vi "Dashboard Main.vi"() -> ()   [LabVIEW 2015]
uses:
  <vilib>/Utility/miscctls.llb/LVRowAndColumnTypeDef.ctl
  <vilib>/event_ctls.llb/eventvkey.ctl
  <vilib>/Rock Robotics/WPI/Dashboard/WPI_DashboardLogging Global.vi
  <vilib>/Rock Robotics/Network Tables/NT Read Numeric Array.vi
  <vilib>/Rock Robotics/Network Tables/NT Read Boolean.vi
  <vilib>/Utility/config.llb/Write Key (String).vi
  <vilib>/Utility/config.llb/Write Key (I32).vi
  <vilib>/Utility/config.llb/NI_LVConfig.lvlib
panel:
  in  "TCP":refnum<k5>
  in  "Rec Mode":enum32{"Stop", "Record", "Playback"}(radio)
  in  "Vision":u16(ring) items=["Camera Off", "USB Camera SW", "USB Camera HW", "IP Camera"]
  out "Camera IP":string
  out "Image Message":string="Timeout in Camera Communications"
  in  "Dashboard Tab":T1(tab)
  out "Waveform Chart":dbl(graph)
  in  "Drive Mode":enum16{"Tank Drive", "Arcade Drive"}(ring)
  in  "Controller Mode":enum16{"X-Box Controller", "Joysticks"}(ring)
  in  "Select Auto":string(combo)
  out "NT Connection":bool
  in  "Camera Settings":T2={"Frame Rate"=30, "Compression"=30, "Size"=1} {"Frame Rate" scale=1.0..30.0; "Size" items=["640x480", "320x240", "160x120"]}
  out "MotorChart R":cluster{"Numeric":dbl, "Numeric":dbl}(graph)
  out "MotorChart L":T3(graph)
  out "MotorSliders R":cluster{"MotorSlide1":dbl, "MotorSlide2":dbl} {"MotorSlide2" scale=-1.0..1.0 scale format="%#_2e"; "MotorSlide1" scale=-1.0..1.0 scale format="%#_2e"}
  out "MotorSliders L":T4 {"MotorSlide4 2" scale=0.0..14.0 scale format="%#_2e"; "MotorSlide2" scale=-1.0..1.0 scale format="%#_2e"; "MotorSlide1" scale=-1.0..1.0 scale format="%#_2e"}
  out "Gyro":dbl(knob) scale=0.0..360.0
  out "JS1 Z":dbl(slide) scale=-1.0..1.0 scale format="%#_2e"
  out "JS1 Graph":cluster{"X":dbl, "Y":dbl}[](graph)
  out "JS1 Buttons":T5
  out "JS2 Z":dbl(slide) scale=-1.0..1.0 scale format="%#_2e"
  out "JS2 Graph":cluster{"X":dbl, "Y":dbl}[](graph)
  out "JS2 Buttons":T5
  out "Mode":T6(ring)=enum."Auto Disabled"
  in  "DB Camera Config":bool
  out "fps":dbl format="%#.1g"
  out "Mbps":dbl format="%#.1g"
  out "Mbps LED":bool
  out "Arm Angle":dbl(knob)
  out "Lower Switch":bool
  out "Upper Switch":bool
  out "Code Version":string
  out "Dashboard Version":string
  in  "DB/String 9":string
  in  "DB/String 8":string
  in  "DB/String 7":string
  in  "DB/String 6":string
  in  "DB/String 5":string
  in  "DB/String 4":string
  in  "DB/String 3":string
  in  "DB/String 2":string
  in  "DB/String 1":string
  in  "DB/String 0":string
  in  "DB/Slider 0":dbl(slide) scale=0.0..5.0
  in  "DB/Slider 1":dbl(slide) scale=0.0..5.0
  in  "DB/Slider 2":dbl(slide) scale=0.0..5.0
  in  "DB/Slider 3":dbl(slide) scale=0.0..5.0
  out "DB/LED 3":bool
  out "DB/LED 2":bool
  out "DB/LED 1":bool
  out "DB/LED 0":bool
  in  "DB/Button 3":bool
  in  "DB/Button 2":bool
  in  "DB/Button 1":bool
  in  "DB/Button 0":bool caption="New Name"
  in  "Test Slider":dbl(slide) scale=0.0..100.0 scale format="%#_3g"
  in  "On/Off":bool caption="Solenoid"
  in  "Test Name":u16(ring) items=["Select the test to run..."]
  in  "Test Tree":string(tree)
  in  "Motor":cluster{"Value":dbl, "Enable":bool} {"Value" scale=-1.0..1.0 scale format="%#_3g"}
  out "Progress":T7 {"Test Progress" scale=0.0..100.0}
  in  "Rev/Fwd":cluster{"Forward":bool, "Reverse":bool}
  in  "Test Ring":u16(ring) items=["Monochrome", "Color"]
  out "Cmd Status":string
  in  "Execute Command":bool
  in  "Command Params":string[][](table)
  in  "Command Selection":i32(listbox)
  in  "CheckList":i32(listbox)
  out "Tree":string(tree)
  out "Camera Image":T8(plugin-control)
  out "Background":bool
  # "Arm Angle"
  # "Left"
  # "Front"
  # "Right"
  # "Arm"
  # "Lower Switch"
  # "Upper Switch"
  # "Autonomous Mode"
  # "Controller Mode"
  # "Battery"
  # "Robot Code Version"
  # "Drive Mode"
  # "Dashboard Code Version"
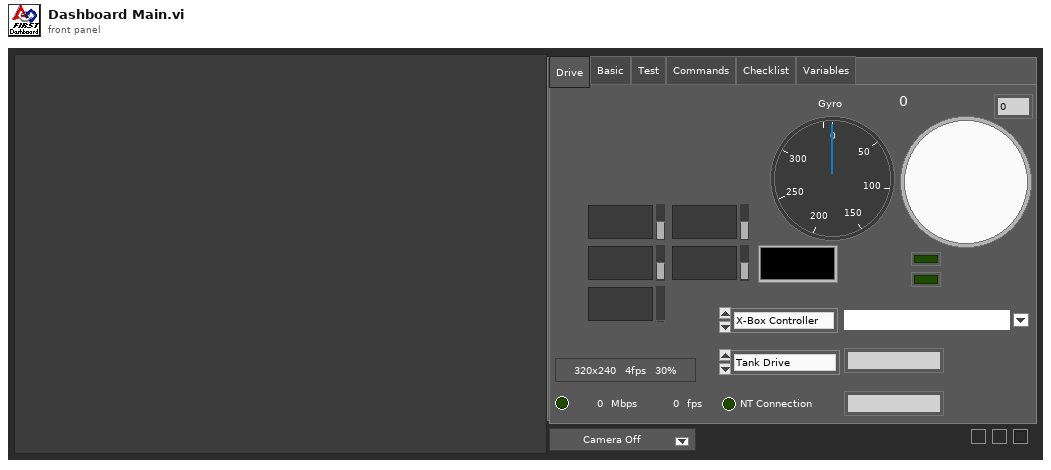
[diagram p1: front panel]
types:
  T1 = enum32{"Drive", "Basic", "Test", "Commands", "Checklist", "Variables"}
  T2 = cluster{"Frame Rate":i32, "Compression":i32, "Size":u16}
  T3 = cluster{"Numeric":dbl, "Numeric":dbl, "Battery V":dbl}
  T4 = cluster{"MotorSlide1":dbl, "MotorSlide2":dbl, "MotorSlide4 2":dbl}
  T5 = cluster{bool, bool, bool, bool, bool, bool, bool, bool, bool, bool, bool, bool}
  T6 = enum8{"Tele-Op Disabled", "Tele-Op Enabled", "Auto Disabled", "Auto Enabled", "Test Disabled", "Test Enabled", "Disconnected", "No Code", "E-Stop"}
  T7 = cluster{"Test Progress":u8, "Test Progress Text":string}
  T8 = typedef "IMAQ Image.ctl" = refnum<image>
  T9 = cluster{"IDs":cluster{"RPC field ID":u16, "Unique ID":u16}, "String":string}
  T10 = enum32{"Drive", "Basic", "Custom", "Test", "Checklist", "Variables"}
  T11 = typedef "Image Type" = u32
  T12 = cluster{"Camera Image":refnum<vi>, "Dashboard Tab":refnum<vi>, "Background":refnum<vi>, "Vision":refnum<vi>, "Rec Mode":refnum<vi>, "Test Slider":refnum<vi>, "On/Off ":refnum<vi>, "Test Ring":refnum<vi>, "Rev/Fwd":refnum<vi>, "Test Name":refnum<vi>, "Motor":refnum<vi>, "Progress":refnum<vi>, "CheckList":refnum<vi>, "Tree":refnum<vi>, "Test Tree":refnum<vi>, "Command Params":refnum<vi>, "Command Selection":refnum<vi>, "Execute Command":refnum<vi>, "Cmd Status":refnum<vi>}
  T13 = cluster{"Error Strings":string, "Disable Counts":cluster{u16, u16}, "Rail Faults":cluster{u16, u16, u16}, "Robot IP":string, "DB Mode":u8, "Event Info":cluster{"Name":string, "Type":u8, "Number":u16, "Replay":u8}, "Camera Addr":string}
  T14 = cluster{"Storage":cluster{"Disk Free":u64, "RAM Block":u32, "RAM free":u32}, "CPU Utilization":cluster{"CPU % ISR":sgl, "CPU % Time Crit":sgl, "CPU % Timed Str":sgl, "CPU % High":sgl, "CPU % Above":sgl, "CPU % Normal":sgl, "CPU % Low":sgl}, "CAN":cluster{"% Bus Utilization":sgl, "Bus Off Cnt":u32, "TX_FIFO Full Cnt":u32, "Receive Error Cnt":u8, "Transmit Error Cnt":u8}, "HID":cluster{"HID Outputs":u32, "Rumble Low":u16, "Rumble High":u16}[]}
  T15 = cluster{"Status bits":cluster{"Test Mode":bool, "Autonomous":bool, "Enabled":bool, "Code Start":bool, "Brownout":bool, "Reserved 2":bool, "Reserved 3":bool, "E-Stop":bool}, "Code Trace":cluster{"Disabled":bool, "TeleOp":bool, "Auto":bool, "Test":bool}, "Controller Type":enum16{"unknown", "cRIO", "roboRio"}, "Code?":enum16{"unknown", "noCode", "code"}, "Battery V":dbl}
  T16 = cluster{"Control Bits":cluster{"TestMode":bool, "Autonomous":bool, "Enabled":bool, "FMS Present":bool, bool, bool, bool, "E-Stop":bool}, "Team Station ":u8, "Countdown":sgl, "Joystick Values":cluster{"Axes":dbl[], "Buttons":bool[], "POVs":i16[]}[]}
  T17 = cluster{"Axes":dbl[], "Buttons":bool[], "POVs":i16[]}[]
  T18 = cluster{"Axes":dbl[], "Buttons":bool[], "POVs":i16[]}
  T19 = cluster{"Buttons[0]":bool, "Buttons[1]":bool, "Buttons[2]":bool, "Buttons[3]":bool, "Buttons[4]":bool, "Buttons[5]":bool, "Buttons[6]":bool, "Buttons[7]":bool, "Buttons[8]":bool, "Buttons[9]":bool, "Buttons[10]":bool, "Buttons[11]":bool}
  T20 = typedef "NI_LVConfig.lvlib/Config Data RefNum.ctl" = refnum<k1>
  T21 = cluster{"Operation":enum16{"Update", "Clear"}, "Color Box":u32}[]
  T22 = typedef "eventvkey.ctl" = enum16{"ASCII", "Enter", "Return", "Shift", "Ctrl", "Alt", "Cmd", "Opt", "Caps", "NumLock", "Clear", "Break", "Up", "Down", "Left", "Right", "Insert", "Delete", "Home", "End", "PageUp", "PageDown", "Escape", "Help", "Pause", "ScrollLock", "F1", "F2", "F3", "F4", "F5", "F6", "F7", "F8", "F9", "F10", "F11", "F12", "F13", "F14", "F15", "F16", "F17", "F18", "F19", "F20", "F21", "F22", "F23", "F24", "Play", "VolumeUp", "VolumeDown", "Mute", "Two Byte Char"}
  T23 = cluster{"Image Size":bool, "Image Type":bool, "Pixel Value":bool, "ROI Information":bool, "Zoom Factor":bool}
  T24 = enum8{"Enabled", "Disabled", "Disabled and Grayed Out"}
  T25 = cluster{"Operation":enum16{"Update", "Clear"}, "Color Box":u32}
  T26 = typedef "LVRowAndColumnTypeDef.ctl" = cluster{"Row":i32, "Column":i32}
  T27 = cluster{"Shift":bool, "Ctrl":bool, "Alt":bool, "Cmd":bool, "Opt":bool}
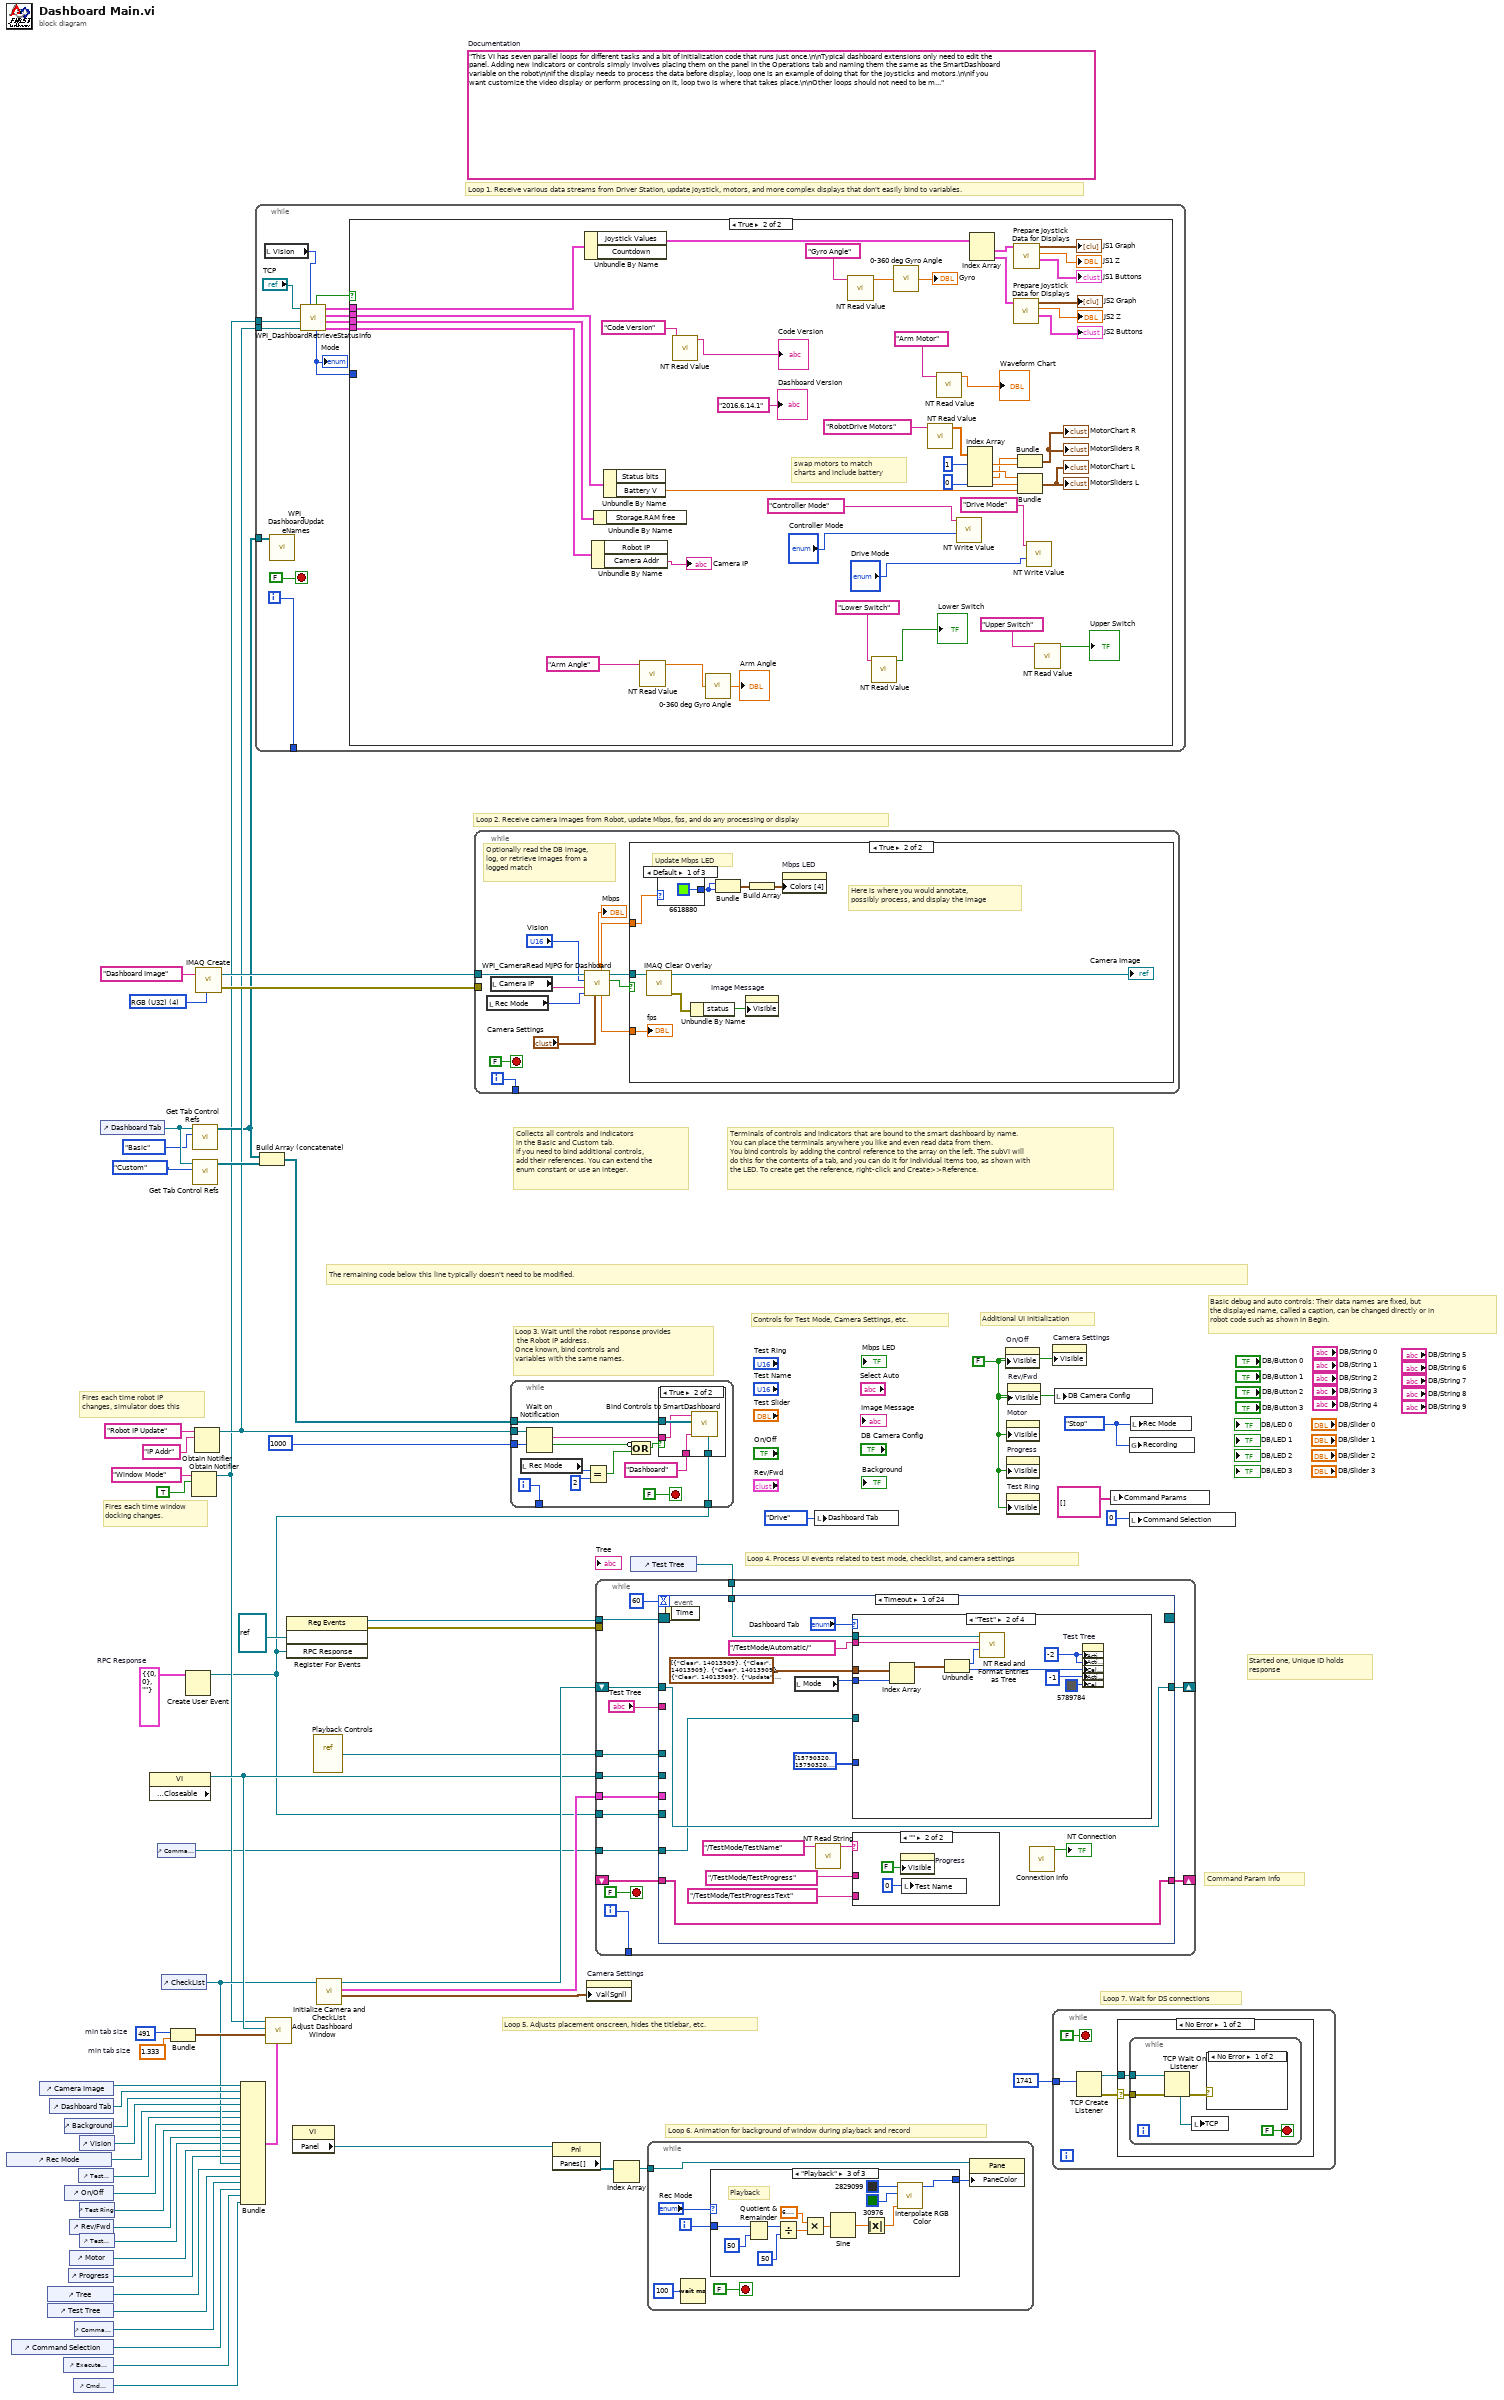
[diagram p0: block diagram]
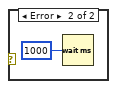
[diagram p2: hidden frame]
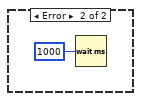
[diagram p3: hidden frame]
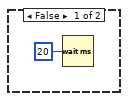
[diagram p4: hidden frame]
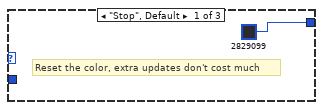
[diagram p5: hidden frame]
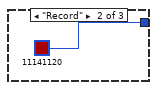
[diagram p6: hidden frame]
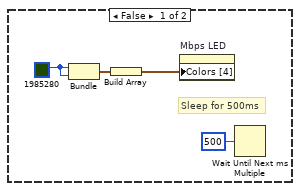
[diagram p8: hidden frame]
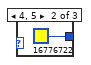
[diagram p9: hidden frame]
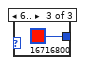
[diagram p10: hidden frame]
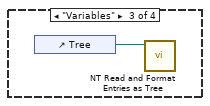
[diagram p12: hidden frame]
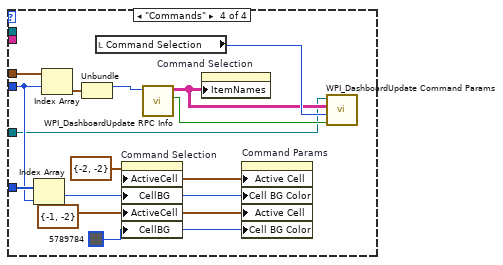
[diagram p13: hidden frame]
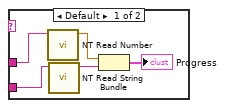
[diagram p14: hidden frame]
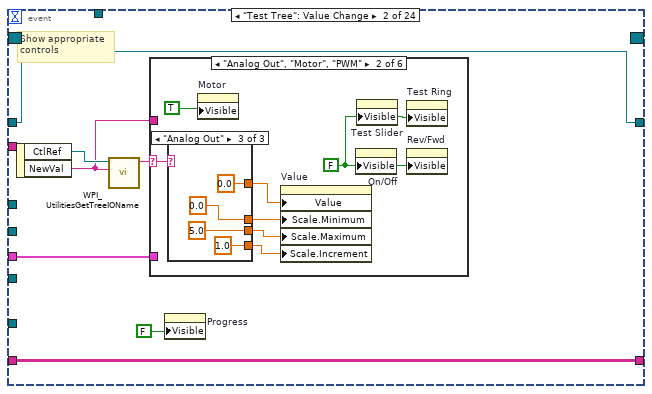
[diagram p15: hidden frame]
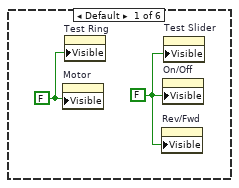
[diagram p16: hidden frame]
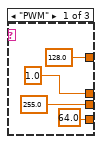
[diagram p17: hidden frame]
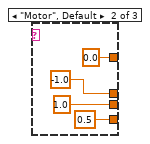
[diagram p18: hidden frame]
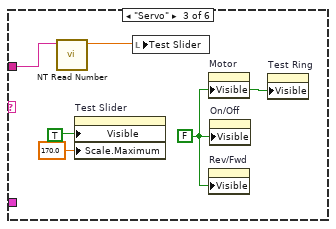
[diagram p19: hidden frame]
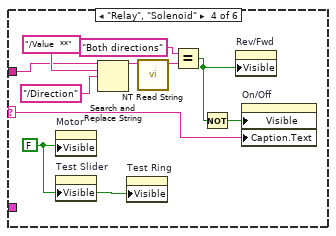
[diagram p20: hidden frame]
diagram:
  w8 = T9 {"IDs"={"RPC field ID"=0, "Unique ID"=0}, "String"=""}  # RPC Response
  w33 = 491  # min tab size
  w32 = 1.333  # min tab size
  w41 = enum32{"Stop", "Record", "Playback"}."Stop" ("Rec Mode")
  w15 = FALSE ("Visible")
  (unwired) "This VI has seven parallel loops for different tasks and a bit of initialization code that runs just once.\n\nTypical dashboard extensions only need to edit the panel. Adding new indicators or controls simply involves placing them on the panel in the Operations tab and naming them the same as the SmartDashboard variable on the robot\n\nIf the display needs to process the data before display, loop one is an example of doing that for the joysticks and motors.\n\nIf you want customize the video display or perform processing on it, loop two is where that takes place.\n\nOther loops should not need to be modified. They are pretty standard, and document the task they perform."  # Documentation
  w61 = T11 4 items=["Grayscale (U8)", "Grayscale (I16)", "Grayscale (SGL)", "Complex (CSG)", "RGB (U32)", "HSL (U32)", "RGB (U64)"] ("Image Type")
  # "Command Param Info"
  # "Started one, Unique ID holds\nresponse"
  # "Loop 7. Wait for DS connections"
  # "Basic debug and auto controls: Their data names are fixed, but\nthe displayed name, called a caption, can be changed directly or in\nrobot code such as shown in Begin."
  # "Controls for Test Mode, Camera Settings, etc."
  # "Additional UI Initialization"
  # "Loop 6. Animation for background of window during playback and record"
  # "Fires each time robot IP\nchanges, simulator does this"
  # "Fires each time window\ndocking changes."
  # "Collects all controls and indicators\nin the Basic and Custom tab.\nIf you need to bind additional controls,\nadd their references. You can extend the\nenum constant or use an integer."
  # "The remaining code below this line typically doesn't need to be modified."
  # "Loop 4. Process UI events related to test mode, checklist, and camera settings"
  # "Terminals of controls and indicators that are bound to the smart dashboard by name.\nYou can place the terminals anywhere you like and even read data from them.\nYou bind controls by adding the control reference to the array on the left. The subVI will\ndo this for the contents of a tab, and you can do it for individual items too, as shown with\nthe LED. To create get the reference, right-click and Create>>Reference."
  # "Loop 3. Wait until the robot response provides\n the Robot IP address.\nOnce known, bind controls and\nvariables with the same names."
  # "Loop 5. Adjusts placement onscreen, hides the titlebar, etc."
  # "Loop 1. Receive various data streams from Driver Station, update joystick, motors, and more complex displays that don't easily bind to variables."
  # "Loop 2. Receive camera images from Robot, update Mbps, fps, and do any processing or display"
  n1 = control-ref of="Rec Mode"() -> (w21:refnum<vi>)
  n2 = control-ref of="Command Selection"() -> (w7:refnum<vi>)
  n3 = control-ref of="Camera Image"() -> (w36:refnum<vi>)
  n4 = control-ref of="Tree"() -> (w25:refnum<vi>)
  n5 = control-ref of="Test Tree"() -> (w24:refnum<vi>)
  n6 = control-ref of="Dashboard Tab"() -> (w35:refnum<vi>)
  n7 = control-ref of="Execute Command"() -> (w9:refnum<vi>)
  n8 = control-ref of="Background"() -> (w30:refnum<vi>)
  n9 = control-ref of="On/Off"() -> (w19:refnum<vi>)
  n10 = control-ref of="Progress"() -> (w16:refnum<vi>)
  n11 = control-ref of="Rev/Fwd"() -> (w17:refnum<vi>)
  n12 = control-ref of="Motor"() -> (w22:refnum<vi>)
  n13 = control-ref of="Cmd Status"() -> (w3:refnum<vi>)
  n14 = control-ref of="Command Params"() -> (w10:refnum<vi>)
  n15 = control-ref of="Test Slider"() -> (w20:refnum<vi>)
  n16 = control-ref of="Vision"() -> (w34:refnum<vi>)
  n17 = control-ref of="Test Ring"() -> (w18:refnum<vi>)
  n18 = control-ref of="Test Name"() -> (w23:refnum<vi>)
  n19 = control-ref of="Dashboard Tab"() -> (w39:refnum<vi>)
  n20 = property class="VI" props=["Front Panel.Closeable"]() -> (reference out=w40:refnum<vi>)  [unwired: 2 in, 2 out]
  n21 = control-ref of="Command Params"() -> (w2:refnum<vi>)
  n22 = control-ref of="CheckList"() -> (w26:refnum<vi>)
  n23 = Bundle("min tab size"=w33, "min tab size"=w32) -> (w31:cluster{"min tab size":i32, "min tab size":dbl})  [unwired: 1 in]
  n24 = Create User Event(user event datatype=w8) -> (user event=w4:refnum<user-event>)  [unwired: 1 in, 1 out]
  n25 = Obtain Notifier(name (unnamed)="Window Mode", notification data type=TRUE) -> (notifier out=w12:refnum<notifier>)  [unwired: 2 in, 2 out]
  n26 = call <vilib>:"Get Tab Control Refs.vi"("Page Index"=T10."Basic" ("Dashboard Tab"), "TabControl in"=w39) -> ("ControlsOnPage"=w13:refnum<vi>[])  [unwired: 9 in]
  n27 = call <vilib>:"Get Tab Control Refs.vi"("Page Index"=T10."Custom" ("Dashboard Tab"), "TabControl in"=w39) -> ("ControlsOnPage"=w38:refnum<vi>[])  [unwired: 9 in]
  n28 = Obtain Notifier(name (unnamed)="Robot IP Update", notification data type="IP Addr" ("name (unnamed)")) -> (notifier out=w14:refnum<notifier>)  [unwired: 2 in, 2 out]
  n29 = call "IMAQ Create"("Image Name"="Dashboard Image", "Image Type"=w61) -> ("New Image"=w59:T8, "error out"=w58:errorcluster)  [unwired: 2 in, 1 out]
  n30 = Bundle("Camera Image"=w36, "Dashboard Tab"=w35, "Background"=w30, "Vision"=w34, "Rec Mode"=w21, "Test Slider"=w20, "On/Off"=w19, "Test Ring"=w18, "Rev/Fwd"=w17, "Test Name"=w23, "Motor"=w22, "Progress"=w16, "CheckList"=w26, "Tree"=w25, "Test Tree"=w24, "Command Params"=w10, "Command Selection"=w7, "Execute Command"=w9, "Cmd Status"=w3) -> (w27:T12)  [unwired: 1 in]
  n31 = while {
    tunnel: [w73] -> _
    tunnel: w14 -> [w67]
    tunnel: w13 -> [w66]
    tunnel: w12 -> [w62]
    i -> [w73]
    stop <- FALSE stop-if-true
    n32 = local read "Vision"() -> (w64:u16)
    n33 = call <vilib>:"WPI_DashboardUpdateNames.vi"("Controls on Tab"=w66) -> ()  [unwired: 11 in]
    n34 = call <vilib>:"WPI_DashboardRetrieveStatusInfo.vi"("Vision"=w64, "Binding Refnum"=w67, "Window Mode Notifier"=w62, "TCP Cnx"="TCP") -> ("Power and Errors"=w68:T13, "Robot Metrics"=w71:T14, "Status Info"=w72:T15, "Control Info"=w69:T16, "Robot Mode"=w65:T6, "Process?"=w70:bool)  [unwired: 2 in]
    "Mode" <- w65
    n35 = case shown="True" w70 {
      tunnel: w72 -> [_ w119]
      tunnel: w71 -> [_ w118]
      tunnel: w69 -> [_ w117]
      tunnel: w68 -> [_ w116]
      tunnel: w65 -> [_ _]
      frame False {
        n36 = Wait (ms)(milliseconds to wait=u32 20) -> ()  [unwired: 1 out]
      }
      frame True {
        # "swap motors to match\ncharts and include battery"
        n37 = Unbundle By Name(w117) -> ("Joystick Values"=w106:T17)  [unwired: 1 out]
        n38 = Unbundle By Name(w116) -> ("Camera Addr"=→"Camera IP":string)  [unwired: 1 out]
        n39 = Unbundle By Name(w118) -> ()  [unwired: 1 out]
        n40 = Unbundle By Name(w119) -> ("Battery V"=w107:dbl)  [unwired: 1 out]
        n41 = call-poly <vilib>:"NT Read Value.vi"("Name"="Arm Angle") -> ("Numeric"=w78:dbl)  [unwired: 9 in, 1 out]
        n42 = call-poly <vilib>:"NT Read Value.vi"("Name"="Code Version") -> ("String"=→"Code Version":string)  [unwired: 9 in, 1 out]
        n43 = call "0-360 deg Gyro Angle.vi"("Raw Angle"=w78) -> ("0-360 deg Angle"=→"Arm Angle":dbl)
        n44 = call-poly <vilib>:"NT Read Value.vi"("Name"="Gyro Angle") -> ("Numeric"=w76:dbl)  [unwired: 9 in, 1 out]
        n45 = call-poly <vilib>:"NT Read Value.vi"("Name"="Lower Switch") -> ("Boolean"=→"Lower Switch":bool)  [unwired: 9 in, 1 out]
        n46 = call "0-360 deg Gyro Angle.vi"("Raw Angle"=w76) -> ("0-360 deg Angle"=→"Gyro":dbl)
        n47 = call-poly <vilib>:"NT Read Value.vi"("Name"="RobotDrive Motors") -> ("Numeric Array"=w95:dbl[])  [unwired: 9 in, 1 out]
        n48 = call-poly <vilib>:"NT Read Value.vi"("Name"="Arm Motor") -> ("Numeric"=→"Waveform Chart":dbl)  [unwired: 9 in, 1 out]
        n49 = call-poly <vilib>:"NT Write Value.vi"("Numeric"="Controller Mode", "Name"="Controller Mode") -> ()  [unwired: 9 in, 1 out]
        n50 = Index Array(array=w95, index #1=1, index #4=0) -> (element #1=w111:dbl, element #2=w112:dbl, element #3=w110:dbl, element #4=w115:dbl)  [unwired: 2 in]
        n51 = Index Array(array=w106) -> (element #1=w105:T18, element #2=w100:T18)  [unwired: 2 in]
        n52 = call "Prepare Joystick Data for Displays.vi"("Joystick Values"=w100) -> ("Buttons"=→"JS2 Buttons":T19, "Z Axis"=→"JS2 Z":dbl, "Cartesian Data"=→"JS2 Graph":cluster{"X axis":dbl, "X axis":dbl}[])  [unwired: 8 in]
        n53 = call "Prepare Joystick Data for Displays.vi"("Joystick Values"=w105) -> ("Buttons"=→"JS1 Buttons":T19, "Z Axis"=→"JS1 Z":dbl, "Cartesian Data"=→"JS1 Graph":cluster{"X axis":dbl, "X axis":dbl}[])  [unwired: 8 in]
        n54 = Bundle("Numeric"=w110, "Numeric"=w111) -> (→"MotorChart R" →"MotorSliders R":cluster{"Numeric":dbl, "Numeric":dbl})  [unwired: 1 in]
        n55 = Bundle("Numeric"=w112, "Numeric"=w115, "Battery V"=w107) -> (→"MotorChart L" →"MotorSliders L":T3)  [unwired: 1 in]
        n56 = call-poly <vilib>:"NT Write Value.vi"("Numeric"="Drive Mode", "Name"="Drive Mode") -> ()  [unwired: 9 in, 1 out]
        n57 = call-poly <vilib>:"NT Read Value.vi"("Name"="Upper Switch") -> ("Boolean"=→"Upper Switch":bool)  [unwired: 9 in, 1 out]
        "Dashboard Version" <- "2016.6.14.1" ("Dashboard Version")
      }
    }
  }
  n58 = Build Array (concatenate)(w13, w38) -> (w37:refnum<vi>[])
  n59 = call "Adjust Dashboard Window.vi"("Sizing Refnums"=w27, "Size Constraints"=w31, "VI"=w40, "WIn Mode"=w12) -> ()  [unwired: 8 in]
  n60 = register-events(refnum<vi> refnum, w4) -> (reference out=w45:refnum<event-registration>, error out=w44:errorcluster)  [unwired: 2 in]
  n61 = property class="VI"() -> ("Panel"=w48:refnum<vi>)  [unwired: 2 in, 2 out]
  n62 = vi-ref "Playback Controls.vi"() -> (w46:refnum<vi>)
  n63 = call "Initialize Camera and CheckList.vi"("ListBox in"=w26) -> ("Cluster"=w52:cluster{"value":i32, "value":i32, "index":i32}, "Array"=w53:cluster{string[]}[], "File Refnum"=w51:T20)  [unwired: 8 in]
  n64 = while {
    tunnel: w59 -> [w128]
    tunnel: w58 -> [_]
    tunnel: [w129] -> _
    i -> [w129]
    stop <- FALSE stop-if-true
    # "Optionally read the DB image,\nlog, or retrieve images from a\nlogged match"
    n65 = local read "Rec Mode"() -> (w123:enum32{"Stop", "Record", "Playback"})
    n66 = local read "Camera IP"() -> (w121:string)
    n67 = call <vilib>:"WPI_CameraRead MJPG for Dashboard.vi"("Camera Settings"="Camera Settings", "Rec Mode"=w123, "Camera IP"=w121, "Camera Mode"="Vision", "Refnum in"=w128) -> ("Active"=w126:bool, "Refnum out"=w127:T8, "FPS"=w125:dbl, "Bandwidth (Mbps)"=w120:dbl)  [unwired: 3 in]
    "Mbps" <- w120
    n68 = case shown="True" w126 {
      tunnel: w127 -> [_ w138]
      tunnel: w120 -> [_ w137]
      tunnel: w125 -> [_ w135]
      frame False {
        w131 = u32 1985280 ("Color Box")
        # "Sleep for 500ms"
        n69 = Bundle("Color Box"=w131, "Color Box"=w131) -> (w133:cluster{"Color Box":u32, "Color Box":u32})  [unwired: 1 out]
        n70 = Build Array(w133) -> (w132:cluster{"Color Box":u32, "Color Box":u32}[])
        n71 = property on="Mbps LED" class="Bool (strict)"("Colors [4]"=w132) -> ()  [unwired: 2 in, 2 out]
        n72 = Wait Until Next ms Multiple(millisecond multiple=u32 500) -> ()  [unwired: 1 out]
      }
      frame True {
        # "Here is where you would annotate,\npossibly process, and display the image"
        # "Update Mbps LED"
        n73 = call "IMAQ Clear Overlay"("Image"=w138) -> ("error out"=w142:errorcluster, "Image Out"=→"Camera Image":T8)  [unwired: 2 in, 7 out]
        n74 = case shown="Default" w137 {
          tunnel: [u32 6618880 ("Color Box") u32 16776722 ("Color Box") u32 16716800 ("Color Box")] -> w139
          frame Default {
          }
          frame 4, 5 {
          }
          frame 6.. {
          }
        }
        n75 = Unbundle By Name(w142) -> ("status"=w143:bool)
        n76 = Bundle("Color Box"=w139, "Color Box"=w139) -> (w141:cluster{"Color Box":u32, "Color Box":u32})  [unwired: 1 out]
        n77 = property on="Image Message" class="Str"("Visible"=w143) -> ()  [unwired: 2 in, 2 out]
        n78 = Build Array(w141) -> (w140:cluster{"Color Box":u32, "Color Box":u32}[])
        n79 = property on="Mbps LED" class="Bool (strict)"("Colors [4]"=w140) -> ()  [unwired: 2 in, 2 out]
        "fps" <- w135
      }
    }
  }
  n80 = while {
    tunnel: w37 -> [w159]
    tunnel: w14 -> [w157]
    tunnel: [w155] -> _
    tunnel: u32 1000 ("milliseconds to wait") -> [w154]
    tunnel: w4 -> [w147]
    i -> [w155]
    stop <- FALSE stop-if-true
    n81 = local read "Rec Mode"() -> (w150:enum32{"Stop", "Record", "Playback"})
    n82 = Wait on Notification(notifier=w157, timeout in ms (-1)=w154) -> (notification=w156:string, timed out?=w152:bool)  [unwired: 2 in, 2 out]
    n83 = Equal?(x=w150, y=u16 2 ("Rec Mode")) -> (x = y?=w151:bool)
    n84 = Compound Arithmetic op=OR(invert w152, w151) -> (w153:bool)
    n85 = case shown="True" w153 {
      tunnel: w159 -> [_ w163]
      tunnel: w156 -> [_ w162]
      tunnel: "Dashboard" -> [_ w161]
      tunnel: w147 -> [_ w160]
      frame False {
      }
      frame True {
        n86 = call <vilib>:"Bind Controls to SmartDashboard.vi"("RPC ref"=w160, "Client Name"=w161, "Bound Control Refs"=w163, "Server IP Address"=w162) -> ()  [unwired: 8 in]
      }
    }
  }
  n87 = property class="Pnl"(reference=w48) -> ("Panes[]"=w49:refnum<vi>[])  [unwired: 1 in, 2 out]
  n88 = property on="Camera Settings" class="Clust (strict)"("Val(Sgnl)"=w52) -> ()  [unwired: 2 in, 2 out]
  n89 = Index Array(array=w49) -> (element=w47:refnum<vi>)  [unwired: 1 in]
  n90 = control-ref of="Test Tree"() -> (w50:refnum<vi>)
  n91 = while {
    tunnel: w53 -> [w175]
    shift-right: [w174] -> _
    shift-left: w51 -> [w173]
    tunnel: [w172] -> _
    tunnel: w50 -> [w171]
    tunnel: w46 -> [w170]
    tunnel: w45 -> [w169]
    tunnel: w44 -> [_]
    tunnel: w40 -> [w168]
    tunnel: w4 -> [w167]
    tunnel: w2 -> [w166]
    shift-right: [w165] -> _
    shift-left: _ -> [w164]
    i -> [w172]
    stop <- FALSE stop-if-true
    n92 = event shown="[0] Timeout" {
      selector: w169 -> [_ _ _ _ _ _ _ _ _ _ _ _ _ _ _ _ _ _ _ _ _ _ _ _]
      dyn-events: [_ _ _ _ _ _ _ _ _ _ _ _ _ _ _ _ _ _ w484 _ _ _ _ _] -> _
      timeout: u32 60 ("milliseconds to wait") -> [_ _ _ _ _ _ _ _ _ _ _ _ _ _ _ _ _ _ _ _ _ _ _ _]
      tunnel: w171 -> [w188 _ _ _ _ _ _ _ _ _ _ _ _ _ _ _ _ _ _ _ _ _ _ _]
      tunnel: "Test Tree" -> [_ _ _ _ _ _ _ _ _ _ _ _ _ w447 w456 w459 w464 w473 _ _ _ _ _ _]
      tunnel: w175 -> [_ w226 _ _ _ _ _ _ _ _ _ w409 w440 _ _ _ _ _ _ _ _ _ _ _]
      tunnel: [w185 w225 w329 w335 w345 w349 w355 w367 w375 w381 w394 w408 w433 w446 w454 w458 w463 w472 w486 w502 w504 w512 w523 w528] -> w174
      tunnel: w173 -> [w185 w225 w329 w335 w345 w349 w355 w367 w375 w381 w394 w407 w433 w446 w454 w458 w463 w472 w486 w502 w504 w512 w523 w528]
      tunnel: w170 -> [_ _ _ _ _ _ _ _ _ _ _ _ _ _ _ _ _ _ w487 _ w507 _ _ _]
      tunnel: w168 -> [_ _ _ _ _ _ _ _ _ _ _ _ _ _ _ _ _ _ w482 _ _ _ _ _]
      tunnel: w167 -> [_ _ _ _ _ _ _ _ _ _ _ _ _ _ _ _ _ _ w478 _ _ _ _ _]
      tunnel: w166 -> [w180 _ _ _ _ _ w353 _ _ _ _ _ _ _ _ _ _ _ _ _ _ _ _ _]
      tunnel: [w179 w224 w328 w334 w344 w350 w351 w361 w372 w380 w393 w406 w432 w445 w453 w457 w462 w471 w477 w500 w503 w508 w516 w529] -> w165
      tunnel: w164 -> [w179 w224 w328 w334 w344 w350 w351 _ _ w380 w393 w406 w432 w445 w453 w457 w462 w471 w477 w500 w503 w508 w516 w529]
      event Timeout {
        n93 = event-data() -> ()  [unwired: 1 in, 1 out]
        n94 = local read "Mode"() -> (w182:T6)
        n95 = call <vilib>:"NT Read String.vi"("Name"="/TestMode/TestName") -> ("String"=w191:string)  [unwired: 9 in, 1 out]
        n96 = case shown="\"Test\"" "Dashboard Tab" {
          tunnel: w188 -> [_ w202 _ _]
          tunnel: "/TestMode/Automatic/" ("Name Pattern") -> [_ w201 _ _]
          tunnel: T21 [{"Operation"=enum."Clear", "Color Box"=14013909}, {"Operation"=enum."Clear", "Color Box"=14013909}, {"Operation"=enum."Clear", "Color Box"=14013909}, {"Operation"=enum."Clear", "Color Box"=14013909}, {"Operation"=enum."Update", "Color Box"=14013909}, {"Operation"=enum."Update", "Color Box"=16777215}, {"Operation"=enum."Clear", "Color Box"=14013909}, {"Operation"=enum."Clear", "Color Box"=14013909}, {"Operation"=enum."Clear", "Color Box"=14013909}] -> [_ w194 _ w211]
          tunnel: w182 -> [_ w193 _ w210]
          tunnel: u32[] [15790320, 15790320, 15790320, 15790320, 16777215, 16777215, 15790320, 15790320, 15790320] -> [_ _ _ w216]
          tunnel: w180 -> [_ _ _ w204]
          frame "Basic", Default {
          }
          frame "Test" {
            w200 = -2 ("Active Item:Row Number")
            n97 = Index Array(array=w194, index=w193) -> (element=w195:T25)
            n98 = Unbundle(w195) -> ("Operation"=w196:enum16{"Update", "Clear"}, "Color Box"=w197:u32)
            n99 = call <vilib>:"NT Read and Format Entries as Tree.vi"("Operation"=w196, "Name Pattern"=w201, "Tree Refnum"=w202) -> ()  [unwired: 7 in, 2 out]
            n100 = property on="Test Tree" class="Tree (strict)"("Active Item Row Number"=w200, "ActiveColNum"=w200, "CellBG"=w197, "Active Item Row Number"=-1 ("Active Item:Row Number"), "CellBG"=u32 5789784 ("Color Box")) -> ()  [unwired: 2 in, 2 out]
          }
          frame "Variables" {
            n101 = control-ref of="Tree"() -> (w203:refnum<vi>)
            n102 = call <vilib>:"NT Read and Format Entries as Tree.vi"("Tree Refnum"=w203) -> ()  [unwired: 9 in, 2 out]
          }
          frame "Commands" {
            w212 = u32 5789784 ("Color Box")
            w213 = T26 {"Row"=-1, "Column"=-2} ("Active Cell:Active Cell")
            w215 = T26 {"Row"=-2, "Column"=-2} ("Active Cell:Active Cell")
            n103 = Index Array(array=w216, index=w210) -> (element=w214:u32)
            n104 = Index Array(array=w211, index=w210) -> (element=w209:T25)
            n105 = Unbundle(w209) -> ("Operation"=w208:enum16{"Update", "Clear"})  [unwired: 1 out]
            n106 = local read "Command Selection"() -> (w207:i32)
            n107 = property on="Command Selection" class="MCListbox (strict)"("ActiveCell"=w215, "CellBG"=w214, "ActiveCell"=w213, "CellBG"=w212) -> ()  [unwired: 2 in, 2 out]
            n108 = call <vilib>:"WPI_DashboardUpdate RPC Info.vi"("Operation"=w208) -> ("update"=w206:bool, "commands"=w205:string[][])  [unwired: 9 in]
            n109 = property on="Command Selection" class="MCListbox (strict)"("ItemNames"=w205) -> ()  [unwired: 2 in, 2 out]
            n110 = property on="Command Params" class="Tbl (strict)"("Active Cell"=w215, "Cell BG Color"=w214, "Active Cell"=w213, "Cell BG Color"=w212) -> ()  [unwired: 2 in, 2 out]
            n111 = call <vilib>:"WPI_DashboardUpdate Command Params.vi"("Update"=w206, "NewVal"=w207, "Commands"=w205, "Param Tbl"=w204) -> ()  [unwired: 7 in, 1 out]
          }
        }
        n112 = case shown="\"\"" w191 {
          tunnel: "/TestMode/TestProgress" ("Name") -> [w218 _]
          tunnel: "/TestMode/TestProgressText" ("Name") -> [w217 _]
          frame Default {
            n113 = call <vilib>:"NT Read Number.vi"("Name"=w218) -> ("Numeric"=w219:dbl)  [unwired: 9 in, 1 out]
            n114 = call <vilib>:"NT Read String.vi"("Name"=w217) -> ("String"=w220:string)  [unwired: 9 in, 1 out]
            n115 = Bundle("Numeric"=w219, "String"=w220) -> (→"Progress":cluster{"Numeric":dbl, "String":string})  [unwired: 1 in]
          }
          frame "" {
            n116 = property on="Progress" class="Clust (strict)"("Visible"=FALSE) -> ()  [unwired: 2 in, 2 out]
            n117 = local write "Test Name"(u16 0) -> ()
          }
        }
        n118 = call <vilib>:"Connextion Info.vi"() -> ("Connected"=→"NT Connection":bool)  [unwired: 10 in, 1 out]
      }
      event "Test Tree": Value Change {
        # "Show appropriate\ncontrols"
        n119 = event-data() -> ("CtlRef"=w229:refnum<vi>, "NewVal"=w227:string)  [unwired: 1 in]
        n120 = call <vilib>:"WPI_UtilitiesGetTreeIOName.vi"("NewVal"=w227, "TreeControl in"=w229) -> ("I/O Name"=w230:string)  [unwired: 9 in]
        n121 = case shown="\"Analog Out\", \"Motor\", \"PWM\"" w230 {
          selector: w230 -> [_ w237 _ w259 w268 _]
          tunnel: w227 -> [_ _ w256 w258 _ w275]
          tunnel: w226 -> [_ _ _ _ _ w274]
          frame Default {
            w232 = FALSE ("Visible")
            w231 = FALSE ("Visible")
            n122 = property on="Motor" class="Clust (strict)"("Visible"=w231) -> ()  [unwired: 2 in, 2 out]
            n123 = property on="Test Ring" class="Ring (strict)"("Visible"=w231) -> ()  [unwired: 2 in, 2 out]
            n124 = property on="Rev/Fwd" class="Clust (strict)"("Visible"=w232) -> ()  [unwired: 2 in, 2 out]
            n125 = property on="On/Off" class="Bool (strict)"("Visible"=w232) -> ()  [unwired: 2 in, 2 out]
            n126 = property on="Test Slider" class="Slide (strict)"("Visible"=w232) -> ()  [unwired: 2 in, 2 out]
          }
          frame "Analog Out", "Motor", "PWM" {
            w238 = FALSE ("Visible")
            n127 = case shown="\"Analog Out\"" w237 {
              tunnel: [1.0 ("Value") -1.0 ("Value") 0.0 ("Value")] -> w236
              tunnel: [255.0 ("Value") 1.0 ("Value") 5.0 ("Value")] -> w235
              tunnel: [128.0 ("Value") 0.0 ("Value") 0.0 ("Value")] -> w234
              tunnel: [64.0 ("Value") 0.5 ("Value") 1.0 ("Value")] -> w233
              frame "PWM" {
              }
              frame "Motor", Default {
              }
              frame "Analog Out" {
              }
            }
            n128 = property on="Motor" class="Clust (strict)"("Visible"=TRUE) -> ()  [unwired: 2 in, 2 out]
            n129 = property on="Value" class="Slide (strict)"("Value"=w234, "Scale.Minimum"=w236, "Scale.Maximum"=w235, "Scale.Increment"=w233) -> ()  [unwired: 2 in, 2 out]
            n130 = property on="On/Off" class="Bool (strict)"("Visible"=w238) -> ()  [unwired: 2 in, 2 out]
            n131 = property on="Test Slider" class="Slide (strict)"("Visible"=w238) -> ()  [unwired: 2 in, 2 out]
            n132 = property on="Test Ring" class="Ring (strict)"("Visible"=w238) -> ()  [unwired: 2 in, 2 out]
            n133 = property on="Rev/Fwd" class="Clust (strict)"("Visible"=w238) -> ()  [unwired: 2 in, 2 out]
          }
          frame "Servo" {
            w254 = FALSE ("Visible")
            n134 = call <vilib>:"NT Read Number.vi"("Name"=w256) -> ("Numeric"=w255:dbl)  [unwired: 9 in, 1 out]
            n135 = property on="Test Slider" class="Slide (strict)"("Visible"=TRUE, "Scale.Maximum"=170.0 ("Scale.Range:Maximum")) -> ()  [unwired: 2 in, 2 out]
            n136 = local write "Test Slider"(w255) -> ()
            n137 = property on="Motor" class="Clust (strict)"("Visible"=w254) -> ()  [unwired: 2 in, 2 out]
            n138 = property on="Rev/Fwd" class="Clust (strict)"("Visible"=w254) -> ()  [unwired: 2 in, 2 out]
            n139 = property on="On/Off" class="Bool (strict)"("Visible"=w254) -> ()  [unwired: 2 in, 2 out]
            n140 = property on="Test Ring" class="Ring (strict)"("Visible"=w254) -> ()  [unwired: 2 in, 2 out]
          }
          frame "Relay", "Solenoid" {
            w257 = FALSE ("Visible")
            n141 = property on="Motor" class="Clust (strict)"("Visible"=w257) -> ()  [unwired: 2 in, 2 out]
            n142 = property on="Test Slider" class="Slide (strict)"("Visible"=w257) -> ()  [unwired: 2 in, 2 out]
            n143 = Search and Replace String(input string=w258, search string="/Value  **", replace string="/Direction") -> (result string=w264:string)  [unwired: 5 in, 3 out]
            n144 = property on="Test Ring" class="Ring (strict)"("Visible"=w257) -> ()  [unwired: 2 in, 2 out]
            n145 = call <vilib>:"NT Read String.vi"("Name"=w264) -> ("String"=w262:string)  [unwired: 9 in, 1 out]
            n146 = Equal?(x="Both directions", y=w262) -> (x = y?=w260:bool)
            n147 = Not(x=w260) -> (.not. x?=w261:bool)
            n148 = property on="Rev/Fwd" class="Clust (strict)"("Visible"=w260) -> ()  [unwired: 2 in, 2 out]
            n149 = property on="On/Off" class="Bool (strict)"("Visible"=w261, "Caption.Text"=w259) -> ()  [unwired: 2 in, 2 out]
          }
          frame "Compressor", "Digital Out" {
            w267 = FALSE ("Visible")
            # "Get direction and finish"
            n150 = property on="Motor" class="Clust (strict)"("Visible"=w267) -> ()  [unwired: 2 in, 2 out]
            n151 = property on="Test Slider" class="Slide (strict)"("Visible"=w267) -> ()  [unwired: 2 in, 2 out]
            n152 = property on="Test Ring" class="Ring (strict)"("Visible"=w267) -> ()  [unwired: 2 in, 2 out]
            n153 = property on="On/Off" class="Bool (strict)"("Visible"=TRUE, "Caption.Text"=w268) -> ()  [unwired: 2 in, 2 out]
            n154 = property on="Rev/Fwd" class="Clust (strict)"("Visible"=FALSE) -> ()  [unwired: 2 in, 2 out]
          }
          frame "Camera" {
            n155 = call <vilib>:"Get Last Path Segment.vi"("String in"=w275) -> ("String out"=w276:string)  [unwired: 10 in]
            n156 = property on="On/Off" class="Bool (strict)"("Visible"=FALSE) -> ()  [unwired: 2 in, 2 out]
            n157 = property on="Motor" class="Clust (strict)"("Visible"=FALSE) -> ()  [unwired: 2 in, 2 out]
            n158 = property on="Rev/Fwd" class="Clust (strict)"("Visible"=FALSE) -> ()  [unwired: 2 in, 2 out]
            n159 = case shown="\"White Balance  **\"" w276 {
              tunnel: w275 -> [w282 w291 w300 w309 w318 _ w324]
              tunnel: w274 -> [w280 w288 w297 w306 w315 _ _]
              frame "Size  **" {
                n160 = Index Array(array=w280) -> (element=w279:cluster{string[]})  [unwired: 1 in]
                n161 = call <vilib>:"NT Read String.vi"("Name"=w282) -> ("String"=w281:string)  [unwired: 9 in, 1 out]
                n162 = Unbundle(w279) -> (w277:string[])
                n163 = Match First String(2:w277, 3:w281) -> (0:w278:i32)  [unwired: 1 out]
                n164 = property on="Test Ring" class="Ring (strict)"("Value"=w278, "Strings []"=w277) -> ()  [unwired: 2 in, 2 out]
                n165 = property on="Test Ring" class="Ring (strict)"("Visible"=TRUE) -> ()  [unwired: 2 in, 2 out]
                n166 = property on="Test Slider" class="Slide (strict)"("Visible"=FALSE) -> ()  [unwired: 2 in, 2 out]
              }
              frame "White Balance  **" {
                n167 = Index Array(array=w288, index=1) -> (element=w289:cluster{string[]})
                n168 = call <vilib>:"NT Read String.vi"("Name"=w291) -> ("String"=w290:string)  [unwired: 9 in, 1 out]
                n169 = Unbundle(w289) -> (w286:string[])
                n170 = Match First String(2:w286, 3:w290) -> (0:w285:i32)  [unwired: 1 out]
                n171 = property on="Test Ring" class="Ring (strict)"("Value"=w285, "Strings []"=w286) -> ()  [unwired: 2 in, 2 out]
                n172 = property on="Test Ring" class="Ring (strict)"("Visible"=TRUE) -> ()  [unwired: 2 in, 2 out]
                n173 = property on="Test Slider" class="Slide (strict)"("Visible"=FALSE) -> ()  [unwired: 2 in, 2 out]
              }
              frame "Exposure  **" {
                n174 = Index Array(array=w297, index=2) -> (element=w298:cluster{string[]})
                n175 = call <vilib>:"NT Read String.vi"("Name"=w300) -> ("String"=w299:string)  [unwired: 9 in, 1 out]
                n176 = Unbundle(w298) -> (w294:string[])
                n177 = Match First String(2:w294, 3:w299) -> (0:w295:i32)  [unwired: 1 out]
                n178 = property on="Test Ring" class="Ring (strict)"("Value"=w295, "Strings []"=w294) -> ()  [unwired: 2 in, 2 out]
                n179 = property on="Test Ring" class="Ring (strict)"("Visible"=TRUE) -> ()  [unwired: 2 in, 2 out]
                n180 = property on="Test Slider" class="Slide (strict)"("Visible"=FALSE) -> ()  [unwired: 2 in, 2 out]
              }
              frame "Exposure Priority  **" {
                n181 = Index Array(array=w306, index=3) -> (element=w307:cluster{string[]})
                n182 = call <vilib>:"NT Read String.vi"("Name"=w309) -> ("String"=w308:string)  [unwired: 9 in, 1 out]
                n183 = Unbundle(w307) -> (w303:string[])
                n184 = Match First String(2:w303, 3:w308) -> (0:w304:i32)  [unwired: 1 out]
                n185 = property on="Test Ring" class="Ring (strict)"("Value"=w304, "Strings []"=w303) -> ()  [unwired: 2 in, 2 out]
                n186 = property on="Test Ring" class="Ring (strict)"("Visible"=TRUE) -> ()  [unwired: 2 in, 2 out]
                n187 = property on="Test Slider" class="Slide (strict)"("Visible"=FALSE) -> ()  [unwired: 2 in, 2 out]
              }
              frame "Color Enable  **" {
                n188 = Index Array(array=w315, index=4) -> (element=w316:cluster{string[]})
                n189 = call <vilib>:"NT Read String.vi"("Name"=w318) -> ("String"=w317:string)  [unwired: 9 in, 1 out]
                n190 = Unbundle(w316) -> (w312:string[])
                n191 = Match First String(2:w312, 3:w317) -> (0:w313:i32)  [unwired: 1 out]
                n192 = property on="Test Ring" class="Ring (strict)"("Value"=w313, "Strings []"=w312) -> ()  [unwired: 2 in, 2 out]
                n193 = property on="Test Ring" class="Ring (strict)"("Visible"=TRUE) -> ()  [unwired: 2 in, 2 out]
                n194 = property on="Test Slider" class="Slide (strict)"("Visible"=FALSE) -> ()  [unwired: 2 in, 2 out]
              }
              frame Default {
                n195 = property on="Test Ring" class="Ring (strict)"("Visible"=FALSE) -> ()  [unwired: 2 in, 2 out]
                n196 = property on="Test Slider" class="Slide (strict)"("Visible"=FALSE) -> ()  [unwired: 2 in, 2 out]
              }
              frame "Brightness  **", "Color Level  **", "Compression  **", "FPS  **", "Sharpness  **" {
                n197 = call <vilib>:"NT Read Number.vi"("Name"=w324) -> ("Numeric"=w323:dbl)  [unwired: 9 in, 1 out]
                n198 = local write "Test Slider"(w323) -> ()
                n199 = property on="Test Slider" class="Slide (strict)"("Visible"=TRUE, "Scale.Maximum"=100.0 ("Scale.Range:Maximum")) -> ()  [unwired: 2 in, 2 out]
                n200 = property on="Test Ring" class="Ring (strict)"("Visible"=FALSE) -> ()  [unwired: 2 in, 2 out]
              }
            }
          }
        }
        n201 = property on="Progress" class="Clust (strict)"("Visible"=FALSE) -> ()  [unwired: 2 in, 2 out]
      }
      event "Test Name": Mouse Enter {
        # "Populate the ring with the list of tests"
        n202 = event-data() -> ()  [unwired: 1 in, 1 out]
        n203 = call <vilib>:"NT Read String Array.vi"("Name"="/TestMode/TestList") -> ("String Array"=w333:string[])  [unwired: 9 in, 1 out]
        n204 = Build Array (concatenate)("Select the test to run...", w333) -> (w332:string[])
        n205 = property on="Test Name" class="Ring (strict)"("Strings []"=w332) -> ()  [unwired: 2 in, 2 out]
      }
      event "Test Name": Value Change {
        w336 = FALSE ("Visible")
        # "Tell the robot the test name to run"
        n206 = event-data() -> ("NewVal"=w340:u16)  [unwired: 1 in]
        n207 = property on="Test Name" class="Ring (strict)"() -> ("Strings []"=w341:string[])  [unwired: 2 in, 2 out]
        n208 = local write "Progress"(T7 {"Test Progress"=0, "Test Progress Text"=""} ("Progress")) -> ()
        n209 = Index Array(array=w341, index=w340) -> (element=w339:string)
        n210 = call <vilib>:"NT Write String.vi"("String"=w339, "Name"="/TestMode/TestName") -> ()  [unwired: 9 in, 1 out]
        n211 = property on="Progress" class="Clust (strict)"("Visible"=TRUE) -> ()  [unwired: 2 in, 2 out]
        n212 = property on="Motor" class="Clust (strict)"("Visible"=w336) -> ()  [unwired: 2 in, 2 out]
        n213 = property on="Test Slider" class="Slide (strict)"("Visible"=w336) -> ()  [unwired: 2 in, 2 out]
        n214 = property on="On/Off" class="Bool (strict)"("Visible"=w336) -> ()  [unwired: 2 in, 2 out]
        n215 = property on="Rev/Fwd" class="Clust (strict)"("Visible"=w336) -> ()  [unwired: 2 in, 2 out]
        n216 = property on="Test Ring" class="Ring (strict)"("Visible"=w336) -> ()  [unwired: 2 in, 2 out]
      }
      event "Select Auto": Mouse Enter {
        # "Populate the combo box with the list of autonomous options"
        n217 = event-data() -> ()  [unwired: 1 in, 1 out]
        n218 = call <vilib>:"NT Read String Array.vi"("Name"="Auto List") -> ("String Array"=w343:string[])  [unwired: 9 in, 1 out]
        n219 = property on="Select Auto" class="CmbBox"("Strings[]"=w343) -> ()  [unwired: 2 in, 2 out]
      }
      event "Select Auto": Value Change {
        # "User modified the Auto Selection. Write to NT variable so robot knows."
        n220 = event-data() -> ("NewVal"=w347:string)  [unwired: 1 in]
        n221 = call <vilib>:"NT Write String.vi"("String"=w347, "Name"="Auto Selector") -> ()  [unwired: 9 in, 1 out]
      }
      event "Command Selection": Value Change {
        # "Get the params and show in table"
        n222 = event-data() -> ("NewVal"=w354:i32)  [unwired: 1 in]
        n223 = property on="Command Selection" class="MCListbox (strict)"() -> ("ItemNames"=w352:string[][])  [unwired: 2 in, 2 out]
        n224 = call <vilib>:"WPI_DashboardUpdate Command Params.vi"("NewVal"=w354, "Commands"=w352, "Param Tbl"=w353) -> ()  [unwired: 8 in, 1 out]
      }
      event "Execute Command": Value Change {
        # "Started one, Unique ID holds\nresponse"
        n225 = event-data() -> ()  [unwired: 1 in, 1 out]
        n226 = property on="Command Selection" class="MCListbox (strict)"() -> ("ItemNames"=w366:string[][])  [unwired: 2 in, 2 out]
        n227 = Index Array(array=w366, index (row)="Command Selection", index (col)=0) -> (element=w364:string)
        n228 = call <vilib>:"Invoke Commands.vi"("Command Params"="Command Params", "Function Name"=w364) -> ("Params"=w360:u8, "Started"=w359:bool)  [unwired: 7 in, 1 out]
        n229 = Array Subset(array="Command Params", length (row)=w360) -> (w361:string[][])  [unwired: 3 in]
        n230 = Select(t="Executing" ("Cmd Status"), s=w359, f="" ("Cmd Status")) -> (s? t:f=→"Cmd Status":string)
      }
      event "Command Selection": Double Click {
        n231 = event-data() -> ("Row"=w376:i32)  [unwired: 1 in]
        n232 = property on="Command Selection" class="MCListbox (strict)"() -> ("ItemNames"=w379:string[][])  [unwired: 2 in, 2 out]
        n233 = local read "Command Params"() -> (w374:string[][])
        n234 = Index Array(array=w379, index (row)=w376, index (col)=0) -> (element=w377:string)
        n235 = call <vilib>:"Invoke Commands.vi"("Command Params"=w374, "Function Name"=w377) -> ("Params"=w373:u8, "Started"=w368:bool)  [unwired: 7 in, 1 out]
        n236 = Array Subset(array=w374, length (row)=w373) -> (w372:string[][])  [unwired: 3 in]
        n237 = Select(t="Executing" ("Cmd Status"), s=w368, f="" ("Cmd Status")) -> (s? t:f=w369:string)
        n238 = local write "Cmd Status"(w369) -> ()
      }
      event "CheckList": Double Click {
        # "Shift clears all"
        # "Update symbols on the listbox"
        n239 = event-data() -> ("PlatMods.Shift"=w382:bool, "Row"=w384:i32)  [unwired: 1 in]
        n240 = case shown="True" w382 {
          tunnel: w384 -> [w388 _]
          tunnel: 1 -> [w387 _]
          frame False {
            n241 = property on="CheckList" class="LstBox (strict)"() -> ("Item Symbols"=w386:i32[])  [unwired: 2 in, 2 out]
            n242 = Replace Array Subset(array=w386, new element=w387, index=w388) -> (w385:i32[])
            n243 = property on="CheckList" class="LstBox (strict)"("Item Symbols"=w385) -> ()  [unwired: 2 in, 2 out]
          }
          frame True {
            w389 = 0 ("Top Row")
            n244 = property on="CheckList" class="LstBox (strict)"() -> ("Number of Rows"=w391:u32)  [unwired: 2 in, 2 out]
            n245 = Initialize Array(0, w391) -> (w390:i32[])
            n246 = property on="CheckList" class="LstBox (strict)"("Top Row"=w389, "Value"=w389, "Item Symbols"=w390) -> ()  [unwired: 2 in, 2 out]
          }
        }
      }
      event "CheckList": Key Down {
        # "Update symbols on the listbox\nLeft and right keys check and uncheck"
        n247 = event-data() -> ("VKey"=w396:T22)  [unwired: 1 in]
        n248 = case shown="\"Left\", \"Right\"" w396 {
          selector: w396 -> [w401 _]
          tunnel: eventvkey."Left" ("VKey") -> [w399 _]
          frame "Left", "Right" {
            n249 = Equal?(x=w399, y=w401) -> (x = y?=w400:bool)
            n250 = Select(t=0, s=w400, f=1) -> (s? t:f=w402:i32)
            n251 = property on="CheckList" class="LstBox (strict)"() -> ("Item Symbols"=w405:i32[])  [unwired: 2 in, 2 out]
            n252 = Replace Array Subset(array=w405, new element=w402, index="CheckList") -> (w404:i32[])
            n253 = property on="CheckList" class="LstBox (strict)"("Item Symbols"=w404) -> ()  [unwired: 2 in, 2 out]
          }
          frame Default {
          }
        }
      }
      event "DB Camera Config": Value Change {
        # "Show or hide the cluster of controls, store in ini file"
        n254 = event-data() -> ("NewVal"=w410:bool)  [unwired: 1 in]
        n255 = case shown="False" w410 {
          tunnel: w409 -> [w419 _]
          tunnel: [w412 w430] -> w408
          tunnel: w407 -> [w411 w430]
          frame False {
            w426 = "Camera"
            w429 = FALSE ("Visible")
            n256 = local read "Camera Settings"() -> (w418:T2)
            n257 = Index Array(array=w419) -> (element=w422:cluster{string[]})  [unwired: 1 in]
            n258 = Unbundle(w418) -> ("Frame Rate"=w417:i32, "Compression"=w416:i32, "Size"=w420:u16)
            n259 = Unbundle(w422) -> (w421:string[])
            n260 = Index Array(array=w421, index=w420) -> (element=w415:string)
            n261 = call-poly <vilib>:"Write Key.vi"("section"=w426, "value"=w415, "key"="Size", "refnum"=w411) -> ("refnum out"=w428:T20)  [unwired: 2 in, 5 out]
            n262 = call-poly <vilib>:"Write Key.vi"("section"=w426, "value"=w417, "key"="FrameRate", "refnum"=w428) -> ("refnum out"=w427:T20)  [unwired: 1 in, 6 out]
            n263 = property on="Camera Settings" class="Clust (strict)"("Visible"=w429) -> ()  [unwired: 2 in, 2 out]
            n264 = local write "DB Camera Config"(w429) -> ()
            n265 = call-poly <vilib>:"Write Key.vi"("section"=w426, "value"=w416, "key"="Compression", "refnum"=w427) -> ("refnum out"=w413:T20)  [unwired: 1 in, 6 out]
            n266 = call <vilib>:"Close Config Data.vi"("refnum"=w413) -> ("file path"=w414:path)  [unwired: 2 in, 8 out]
            n267 = call <vilib>:"Open Config Data.vi"("configuration file path"=w414) -> ("refnum"=w412:T20)  [unwired: 8 in, 2 out]
          }
          frame True {
            n268 = property on="Camera Settings" class="Clust (strict)"("Visible"=TRUE) -> ()  [unwired: 2 in, 2 out]
          }
        }
      }
      event "Camera Settings": Value Change {
        # "Update summary string when any elements of DB camera change"
        n269 = event-data() -> ("NewVal"=w444:T2)  [unwired: 1 in]
        n270 = Index Array(array=w440) -> (element=w439:cluster{string[]})  [unwired: 1 in]
        n271 = Unbundle(w444) -> ("Frame Rate"=w435:i32, "Compression"=w434:i32, "Size"=w437:u16)
        n272 = Unbundle(w439) -> (w438:string[])
        n273 = Index Array(array=w438, index=w437) -> (element=w436:string)
        n274 = Format Into String(format string="%s   %dfps   %d%%", w436, w435, w434) -> (resulting string=w441:string)  [unwired: 2 in, 1 out]
        n275 = Build Array(w441) -> (w442:string[])
        n276 = property on="DB Camera Config" class="Bool (strict)"("Strings [4]"=w442) -> ()  [unwired: 2 in, 2 out]
      }
      event "Motor.Enable": Value Change {
        # "When the test mode otor enable helper is set, update that\ntree row item's value"
        n277 = event-data() -> ("NewVal"=w451:bool)  [unwired: 1 in]
        n278 = Unbundle("Motor") -> ("Value"=w450:dbl)  [unwired: 1 out]
        n279 = Select(t=w450, s=w451, f=0.0) -> (s? t:f=w448:dbl)
        n280 = call <vilib>:"NT Write Number.vi"("Numeric"=w448, "Name"=w447) -> ()  [unwired: 9 in, 1 out]
      }
      event "Test Slider": Value Change {
        # "When the test mode slider helper is set, update that\ntree row item's value"
        n281 = event-data() -> ("NewVal"=w455:dbl)  [unwired: 1 in]
        n282 = call <vilib>:"NT Write Number.vi"("Numeric"=w455, "Name"=w456) -> ()  [unwired: 9 in, 1 out]
      }
      event "On/Off": Value Change {
        # "When the test mode on/off helper value is set, update that\ntree row item's value"
        n283 = event-data() -> ("NewVal"=w461:bool)  [unwired: 1 in]
        n284 = Boolean To (0,1)(Boolean=w461) -> (0, 1=w460:i16)
        n285 = call <vilib>:"NT Write Number.vi"("Numeric"=w460, "Name"=w459) -> ()  [unwired: 9 in, 1 out]
      }
      event "Rev/Fwd": Value Change {
        # "When the test mode helper value for relays is set, update that\ntree row item's value"
        n286 = event-data() -> ("NewVal.Forward"=w470:bool, "NewVal.Reverse"=w469:bool)  [unwired: 1 in]
        n287 = Boolean To (0,1)(Boolean=w470) -> (0, 1=w466:i16)
        n288 = Boolean To (0,1)(Boolean=w469) -> (0, 1=w468:i16)
        n289 = Negate(x=w468) -> (-x=w467:i16)
        n290 = Add(x=w466, y=w467) -> (x+y=w465:i16)
        n291 = call <vilib>:"NT Write Number.vi"("Numeric"=w465, "Name"=w464) -> ()  [unwired: 9 in, 1 out]
      }
      event "Test Ring": Value Change {
        # "When a test mode helper value is selected from the ring,\nset the tree item's variable to the string value"
        n292 = event-data() -> ("NewVal"=w475:u16)  [unwired: 1 in]
        n293 = property on="Test Ring" class="Ring (strict)"() -> ("Strings []"=w476:string[])  [unwired: 2 in, 2 out]
        n294 = Index Array(array=w476, index=w475) -> (element=w474:string)
        n295 = call <vilib>:"NT Write String.vi"("String"=w474, "Name"=w473) -> ()  [unwired: 9 in, 1 out]
      }
      event "Rec Mode": Value Change {
        # "Update globals for recording mode and path to read log from.\nClear when logging and let NetworkTables set path for vision to\nuse."
        n296 = event-data() -> ("NewVal"=w488:enum32{"Stop", "Record", "Playback"})  [unwired: 1 in]
        n297 = global write "WPI_DashboardLogging Global.vi" "Logging Filename"(path "") -> ()
        n298 = global write "WPI_DashboardLogging Global.vi" "Recording"(w488) -> ()
        n299 = case shown="\"Playback\"" w488 {
          tunnel: w487 -> [_ w490 w499]
          tunnel: [_ _ w498] -> w484
          tunnel: [_ _ w497] -> _
          tunnel: w482 -> [_ _ w495]
          tunnel: cluster{i32, i32} {-250, 170} -> [_ _ w494]
          tunnel: [_ _ T23 {"Image Size"=TRUE, "Image Type"=TRUE, "Pixel Value"=TRUE, "ROI Information"=TRUE, "Zoom Factor"=FALSE} ("Image Information Shown:All Elements")] -> w480
          tunnel: [_ _ TRUE ("Zoom Factor")] -> w479
          tunnel: w478 -> [_ _ w491]
          frame Default {
          }
          frame "Stop", "Record" {
            # "Place Window too"
            n300 = invoke class="VI" method="FP.Close"(reference=w490) -> (reference out=w489:refnum<vi>)  [unwired: 2 in, 2 out]
            n301 = invoke class="VI" method="Abort VI"(reference=w489) -> ()  [unwired: 2 in, 3 out]
          }
          frame "Playback" {
            n302 = call "Open Playback Panel.vi"("Offset"=w494, "DB VI Ref"=w495, "Playback in"=w499) -> ("Playback out"=w496:refnum<vi>)  [unwired: 8 in]
            n303 = register-events(w496, w491) -> (reference out=w498:refnum<event-registration>, error out=w497:errorcluster)  [unwired: 2 in]
          }
        }
        n304 = property on="Camera Image" class="ImageControl"("Image Information Shown"=w480, "Image Information Visible"=w479) -> ()  [unwired: 2 in, 2 out]
        n305 = call <vilib>:"WPI_DashboardNT Log FieldName Cache.vi"("Operation"=enum16{"Lookup/Add", "Index", "Clear"}."Clear") -> ()  [unwired: 8 in, 3 out]
      }
      event Panel Close {
        w501 = enum32{"Stop", "Record", "Playback"}."Stop" ("Rec Mode")
        # "Playback window has been closed, abort"
        n306 = event-data() -> ()  [unwired: 1 in, 4 out]
        n307 = local write "Rec Mode"(w501) -> ()
        n308 = global write "WPI_DashboardLogging Global.vi" "Recording"(w501) -> ()
      }
      event Panel Close {
        # "Abort playback window and ourself"
        n309 = event-data() -> ()  [unwired: 1 in, 4 out]
        n310 = invoke class="VI" method="FP.Close"(reference=w507) -> (reference out=w506:refnum<vi>)  [unwired: 2 in, 2 out]
        n311 = invoke class="VI" method="Abort VI"(reference=w506) -> (error out=w505:errorcluster)  [unwired: 2 in, 2 out]
        n312 = invoke class="VI" method="Abort VI"(error in=w505) -> ()  [unwired: 2 in, 3 out]
      }
      event User Event {
        n313 = event-data() -> ("IDs"=w515:cluster{"RPC field ID":u16, "Unique ID":u16}, "String"=w514:string)  [unwired: 1 in]
        n314 = Bundle("IDs"=w515, "String"=w514) -> (w513:T9)  [unwired: 1 in]
        n315 = call <vilib>:"Retrieve RPC Response.vi"("RPC Response"=w513) -> ("Output"=w510:string[][])  [unwired: 10 in]
        n316 = Build Array (concatenate)(w508, w510) -> (w509:string[][])
        n317 = local write "Command Params"(w509) -> ()
        n318 = local write "Cmd Status"("" ("Cmd Status")) -> ()
      }
      event "Vision": Value Change {
        # "Enable/Disable Compression slider.\nHW USB is hard-coded into the camera"
        n319 = event-data() -> ("NewVal"=w522:u16)  [unwired: 1 in]
        n320 = Equal?(x=w522, y=u32 2 ("milliseconds to wait")) -> (x = y?=w520:bool)
        n321 = Select(t=T24."Disabled and Grayed Out" ("Disabled"), s=w520, f=T24."Enabled" ("Disabled")) -> (s? t:f=w517:T24)
        n322 = property on="Compression" class="Slide (strict)"("DisabledEnum"=w517) -> ()  [unwired: 2 in, 2 out]
      }
      event "Tree": Double Click {
        n323 = event-data() -> ("PlatMods"=w527:T27, "Tag"=w526:string)  [unwired: 1 in]
        n324 = Unbundle(w527) -> ("Shift"=w525:bool)  [unwired: 4 out]
        n325 = Not(x=w525) -> (.not. x?=w524:bool)
        n326 = call <vilib>:"NT Update Persistence.vi"("Persistence"=w524, "Name"=w526) -> ()  [unwired: 9 in, 1 out]
      }
    }
  }
  n327 = while {
    tunnel: w47 -> [w531]
    i -> [w534]
    stop <- FALSE stop-if-true
    n328 = Wait (ms)(milliseconds to wait=u32 100) -> ()  [unwired: 1 out]
    n329 = case shown="\"Playback\"" "Rec Mode" {
      tunnel: w534 -> [_ _ w549]
      tunnel: [u32 2829099 ("Base Color") u32 11141120 ("Target Color") w538] -> w530
      frame "Stop", Default {
        # "Reset the color, extra updates don't cost much"
      }
      frame "Record" {
      }
      frame "Playback" {
        # "Playback"
        n330 = Quotient & Remainder(x=w549, y=u32 50 ("milliseconds to wait")) -> (x-y*floor(x/y)=w545:u32)  [unwired: 1 out]
        n331 = Divide(x=w545, y=u32 50 ("milliseconds to wait")) -> (x/y=w542:dbl)
        n332 = Multiply(x=6.283185307179586, y=w542) -> (x*y=w547:dbl)
        n333 = Sine(x=w547) -> (sin(x)=w546:dbl)
        n334 = Absolute Value(x=w546) -> (abs(x)=w539:dbl)
        n335 = call "Interpolate RGB Color.vi"("Proportion"=w539, "Target Color"=u32 30976, "Base Color"=u32 2829099) -> ("Result Color"=w538:u32)  [unwired: 8 in]
      }
    }
    n336 = property class="Pane"(reference=w531, "PaneColor"=w530) -> ()  [unwired: 1 in, 2 out]
  }
  n337 = local write "Dashboard Tab"(T1."Drive" ("Dashboard Tab")) -> ()
  n338 = property on="On/Off" class="Bool (strict)"("Visible"=w15) -> ()  [unwired: 2 in, 2 out]
  n339 = property on="Motor" class="Clust (strict)"("Visible"=w15) -> ()  [unwired: 2 in, 2 out]
  n340 = property on="Progress" class="Clust (strict)"("Visible"=w15) -> ()  [unwired: 2 in, 2 out]
  n341 = property on="Test Ring" class="Ring (strict)"("Visible"=w15) -> ()  [unwired: 2 in, 2 out]
  n342 = property on="Rev/Fwd" class="Clust (strict)"("Visible"=w15) -> ()  [unwired: 2 in, 2 out]
  n343 = property on="Camera Settings" class="Clust (strict)"("Visible"=w15) -> ()  [unwired: 2 in, 2 out]
  n344 = while {
    tunnel: u16 1741 ("timeout ms (25000)") -> [w551]
    stop <- FALSE stop-if-true
    n345 = TCP Create Listener(10:w551) -> (0:w550:errorcluster, 3:w552:refnum<k5>)  [unwired: 4 in, 1 out]
    n346 = case shown="No Error" w550 {
      selector: w550 -> [w554 _]
      tunnel: w552 -> [w555 _]
      frame No Error {
        n347 = while {
          tunnel: w555 -> [w558]
          tunnel: w554 -> [w557]
          stop <- FALSE stop-if-true
          n348 = TCP Wait On Listener(8:w557, 11:w558) -> (0:w559:errorcluster, 4:w560:refnum<k5>)  [unwired: 2 in, 3 out]
          n349 = local write "TCP"(w560) -> ()
          n350 = case shown="No Error" w559 {
            frame No Error {
            }
            frame Error {
              n351 = Wait (ms)(milliseconds to wait=u32 1000) -> ()  [unwired: 1 out]
            }
          }
        }
      }
      frame Error {
        n352 = Wait (ms)(milliseconds to wait=u32 1000) -> ()  [unwired: 1 out]
      }
    }
  }
  n353 = local write "DB Camera Config"(w15) -> ()
  n354 = local write "Command Params"(string[][] [] ("Command Params")) -> ()
  n355 = global write "WPI_DashboardLogging Global.vi" "Recording"(w41) -> ()
  n356 = local write "Command Selection"(u16 0 ("milliseconds to wait")) -> ()
  n357 = local write "Rec Mode"(w41) -> ()
